vi "Open_USB.vi"(8 "entrée d'erreur":errorcluster caption="entrée d'erreur (pas d'erreur)", 9 "Timeout (0)":u32, 10 "Access Mode":T1 items=["VISA Defaults"=0, "Exclusive Lock"=1, "Load Configured Settings"=4], 11 "Nom de ressource VISA":refnum<visa-resource-name>) -> (0 "error out":errorcluster, 3 "Nom de ressource VISA ouverte":refnum<visa-resource-name>)   [LabVIEW 2014]
uses:
  <vilib>/Instr/_visa.llb/VISA Open Access Mode.ctl
  <vilib>/Instr/_visa.llb/Select Event Type.ctl
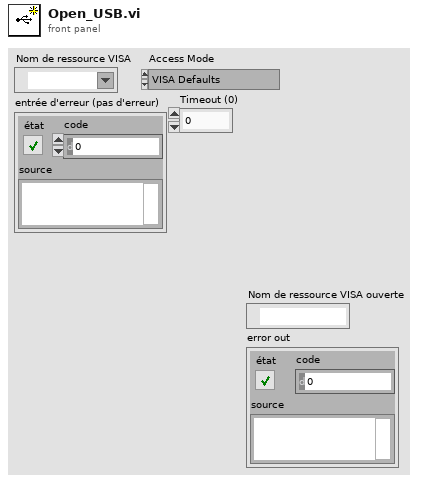
[diagram p1: front panel]
types:
  T1 = typedef "VISA Open Access Mode.ctl" = u32
  T2 = typedef "Select Event Type.ctl" = u32
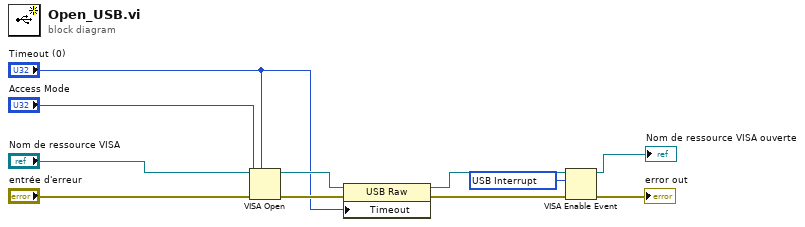
[diagram p0: block diagram]
diagram:
  w11 = T2 1073684535 items=["Service Request"=1073684491, "Trigger"=3221168138, "Clear"=1073684493, "VXI Signal"=1073684512, "VXI/VME Interrupt"=3221168161, "VXI/VME Sysfail"=1073684509, "VXI/VME Sysreset"=1073684510, "GPIB-CIC"=1073684498, "GPIB-Talk"=1073684499, "GPIB-Listen"=1073684500, "PXI Interrupt"=1073684514, "Serial Break"=1073684515, "Serial TermChar"=1073684516, "Serial CTS"=1073684521, "Serial DSR"=1073684522, "Serial DCD"=1073684524, "Serial RI"=1073684526, "Serial Character"=1073684533, "USB Interrupt"=1073684535, "All Enabled"=1073709055] ("Event Type")
  n1 = VISA Open(timeout (0)="Timeout (0)", access mode="Access Mode", error in (no error)="entrée d'erreur", VISA resource name="Nom de ressource VISA") -> (VISA resource name=w5:refnum<visa-resource-name>, error out=w4:errorcluster)  [unwired: 1 in]
  n2 = property class="USB Raw"(reference=w5, error in=w4, "Timeout"="Timeout (0)") -> (reference out=w2:refnum<visa-resource-name>, error out=w3:errorcluster)
  n3 = VISA Enable Event(8:w3, 10:w11, 11:w2) -> (0:→"error out":errorcluster, 3:→"Nom de ressource VISA ouverte":refnum<visa-resource-name>)  [unwired: 1 in]
